vi "Configure Trigger (LIN).vi"(0 "VISA resource name":refnum<visa-resource-name>, 5 "Trigger Source (9: Bus 1)":u16(ring)=9 items=["Bus 1"=9, "Bus 2"=10, "Bus 3"=11, "Bus 4"=12], 7 "Condition (0: Sync field)":u16(ring) items=["Sync Field", "Identifier", "Data", "ID and data", "Wake up", "Sleep", "Error"], 9 "Data":T1={"Data Size (8)"=8, "Data Value (XXXXXXXX)"="XXXXXXXX", "Data Upper Word Value (XXXXXXXX)"="XXXXXXXX", "Data Qualifier (0: Less than)"=0, "Error Type (0: Sync)"=0, "Identifier Value (XXXXXXXX)"="XXXXXXXX"} {"Error Type (0: Sync)" items=["Sync", "Parity", "Checksum", "Header time", "Response time", "Frame time"]; "Data Qualifier (0: Less than)" items=["Less than", "More than", "Equal", "Unequal", "Less equal", "More equal", "In range", "Out of range"]}, 11 "error in (no error)":errorcluster) -> (4 "VISA resource name out":refnum<visa-resource-name>, 15 "error out":errorcluster)   [LabVIEW 2017, in "Scope.lvlib" / "Tektronix DPO MSO 2000 4000 Series.lvlib"]
doc: "Configures Audio trigger settings for an oscilloscope."
uses:
  Tektronix DPO MSO 2000 4000 Series.lvlib
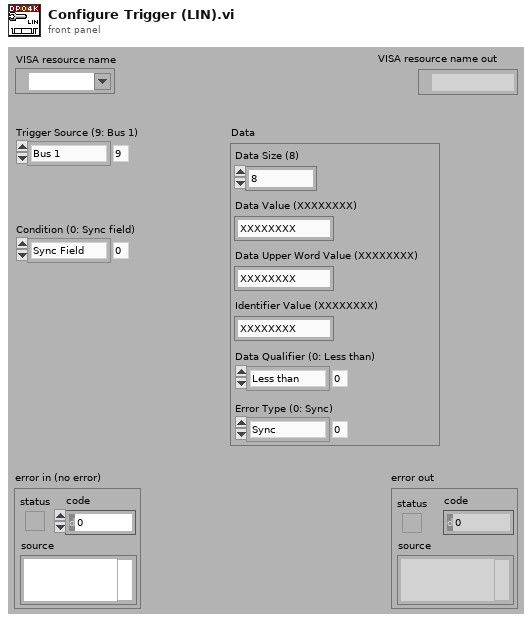
[diagram p1: front panel]
types:
  T1 = cluster{"Data Size (8)":i32, "Data Value (XXXXXXXX)":string, "Data Upper Word Value (XXXXXXXX)":string, "Data Qualifier (0: Less than)":u16, "Error Type (0: Sync)":u16, "Identifier Value (XXXXXXXX)":string}
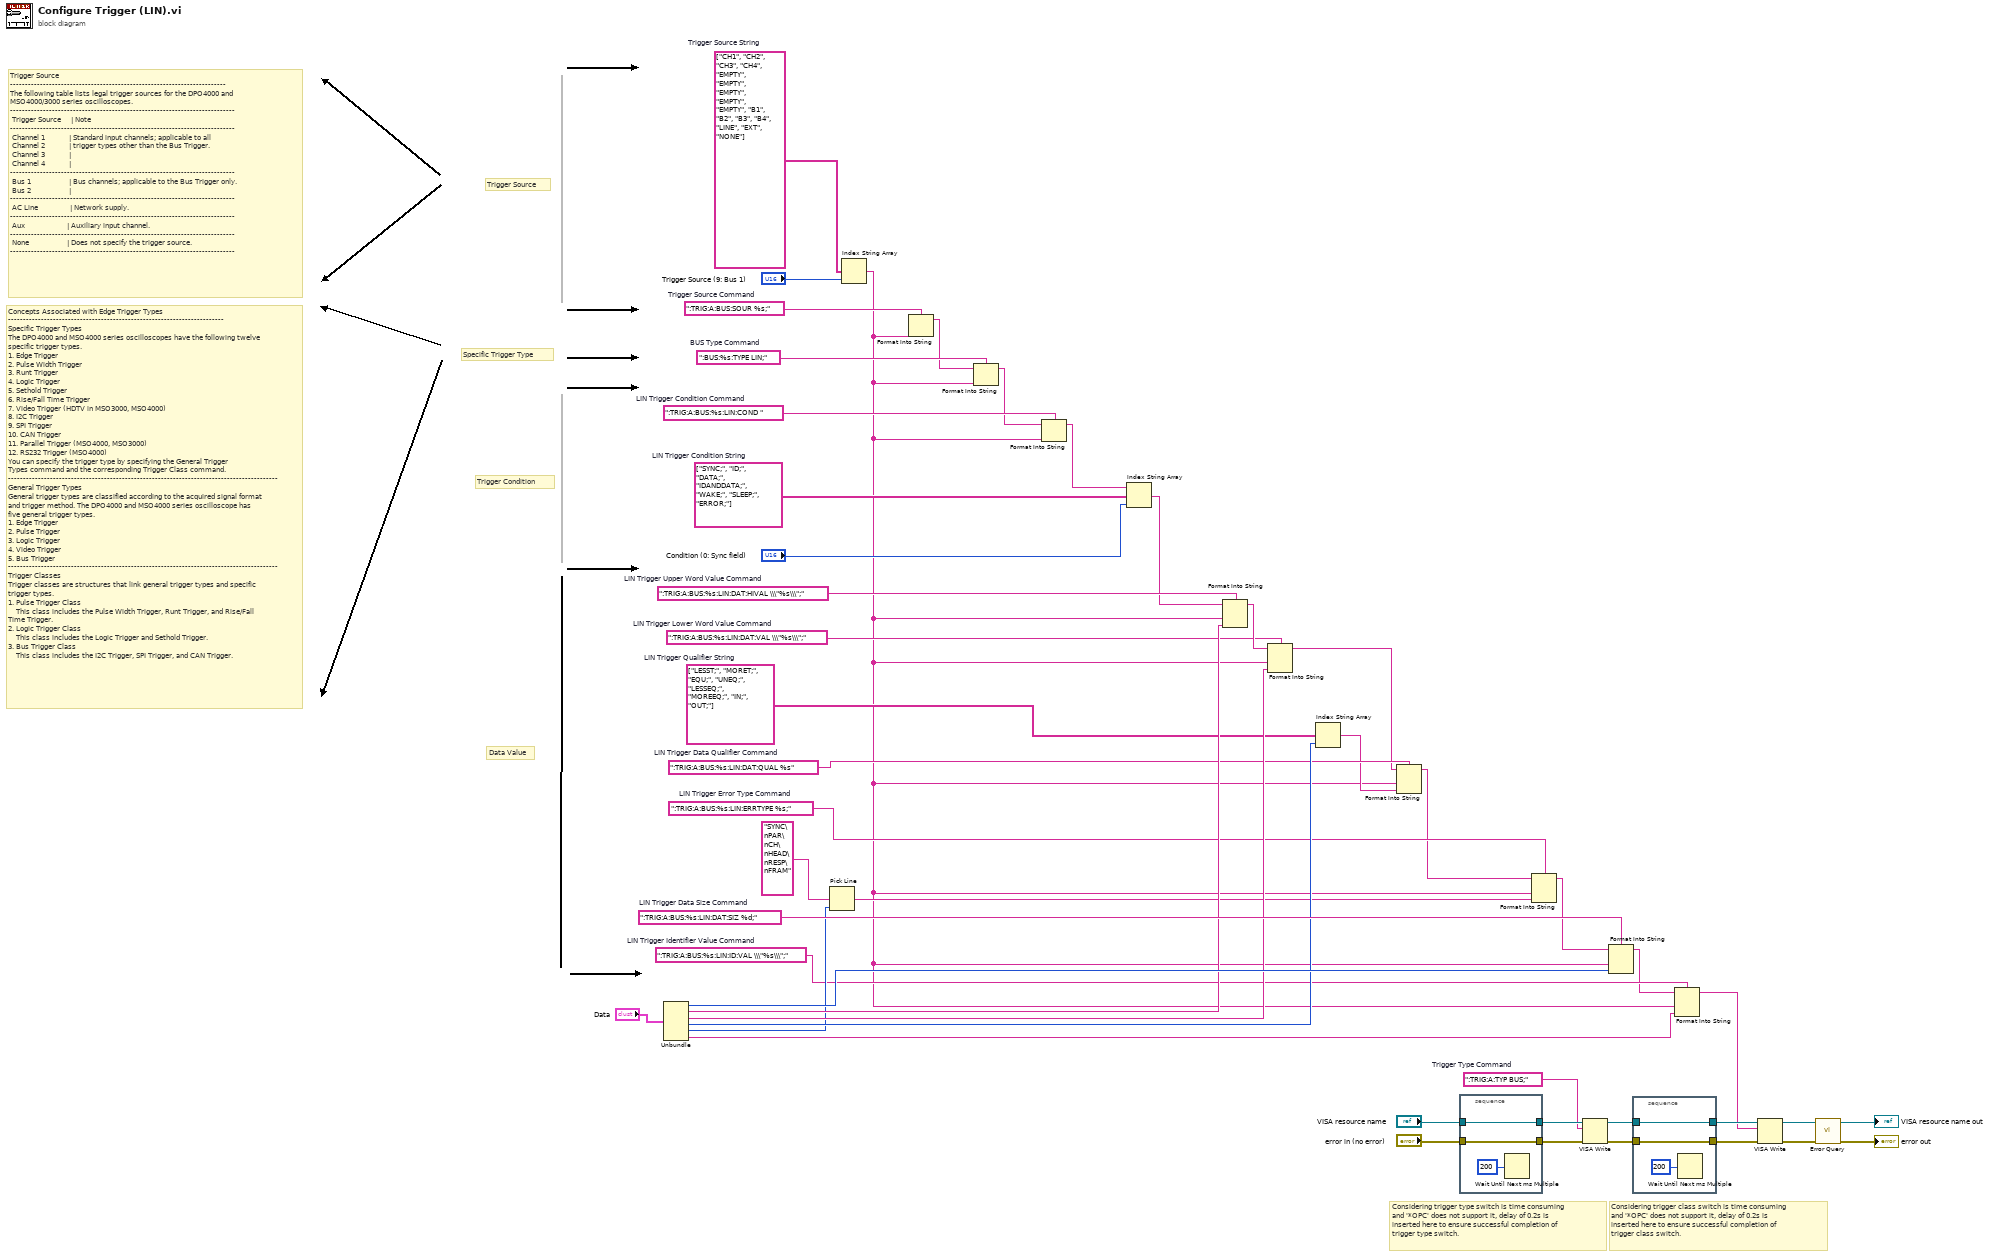
[diagram p0: block diagram]
diagram:
  w5 = ":TRIG:A:BUS:%s:LIN:ID:VAL \\\"%s\\\";"  # LIN Trigger Identifier Value Command
  w8 = ":TRIG:A:BUS:%s:LIN:ERRTYPE %s;"  # LIN Trigger Error Type Command
  w13 = ":TRIG:A:BUS:%s:LIN:DAT:QUAL %s"  # LIN Trigger Data Qualifier Command
  w15 = string[] ["LESST;", "MORET;", "EQU;", "UNEQ;", "LESSEQ;", "MOREEQ;", "IN;", "OUT;"]  # LIN Trigger Qualifier String
  w17 = ":TRIG:A:BUS:%s:LIN:DAT:VAL \\\"%s\\\";"  # LIN Trigger Lower Word Value Command
  w29 = string[] ["CH1", "CH2", "CH3", "CH4", "EMPTY", "EMPTY", "EMPTY", "EMPTY", "EMPTY", "B1", "B2", "B3", "B4", "LINE", "EXT", "NONE"]  # Trigger Source String
  w28 = ":TRIG:A:BUS:SOUR %s;"  # Trigger Source Command
  w36 = ":TRIG:A:TYP BUS;"  # Trigger Type Command
  w42 = ":TRIG:A:BUS:%s:LIN:DAT:SIZ %d;"  # LIN Trigger Data Size Command
  w43 = ":TRIG:A:BUS:%s:LIN:DAT:HIVAL \\\"%s\\\";"  # LIN Trigger Upper Word Value Command
  w45 = string[] ["SYNC;", "ID;", "DATA;", "IDANDDATA;", "WAKE;", "SLEEP;", "ERROR;"]  # LIN Trigger Condition String
  w47 = ":TRIG:A:BUS:%s:LIN:COND "  # LIN Trigger Condition Command
  w27 = ":BUS:%s:TYPE LIN;"  # BUS Type Command
  # "Concepts Associated with Edge Trigger Types\n------------------------------------------------------------------------\nSpecific Trigger Types\nThe DPO4000 and MSO4000 series oscilloscopes have the following twelve specific trigger types.\n1. Edge Trigger\n2. Pulse Width Trigger\n3. Runt Trigger\n4. Logic Trigger\n5. Sethold Trigger\n6. Rise/Fall Time Trigger\n7. Video Trigger (HDTV in MSO3000, MSO4000)\n8. I2C Trigger\n9. SPI Trigger\n10. CAN Trigger\n11. Parallel Trigger (MSO4000, MSO3000)\n12. RS232 Trigger (MSO4000)\nYou can specify the trigger type by specifying the General Trigger \nTypes command and the corresponding Trigger Class command.\n------------------------------------------------------------------------------------------\nGeneral Trigger Types \nGeneral trigger types are classified according to the acquired signal format and trigger method. The DPO4000 and MSO4000 series oscilloscope has five general trigger types.\n1. Edge Trigger\n2. Pulse Trigger\n3. Logic Trigger\n4. Video Trigger\n5. Bus Trigger\n------------------------------------------------------------------------------------------\nTrigger Classes\nTrigger classes are structures that link general trigger types and specific trigger types.\n1. Pulse Trigger Class\n    This class includes the Pulse Width Trigger, Runt Trigger, and Rise/Fall Time Trigger.\n2. Logic Trigger Class\n    This class includes the Logic Trigger and Sethold Trigger.\n3. Bus Trigger Class\n    This class includes the I2C Trigger, SPI Trigger, and CAN Trigger."
  # "Trigger Source\n------------------------------------------------------------------------\nThe following table lists legal trigger sources for the DPO4000 and MSO4000/3000 series oscilloscopes.\n---------------------------------------------------------------------------\n Trigger Source     | Note                                                           \n---------------------------------------------------------------------------\n Channel 1            | Standard input channels; applicable to all      \n Channel 2            | trigger types other than the Bus Trigger.         \n Channel 3            |     \n Channel 4            |\n---------------------------------------------------------------------------\n Bus 1                   | Bus channels; applicable to the Bus Trigger only.\n Bus 2                   | \n---------------------------------------------------------------------------\n AC Line                | Network supply.\n---------------------------------------------------------------------------\n Aux                     | Auxiliary input channel.\n---------------------------------------------------------------------------\n None                   | Does not specify the trigger source.\n---------------------------------------------------------------------------"
  # "Data Value"
  # "Trigger Condition"
  # "Specific Trigger Type"
  # "Trigger Source"
  # "Considering trigger class switch is time consuming\nand '*OPC' does not support it, delay of 0.2s is \ninserted here to ensure successful completion of\ntrigger class switch."
  # "Considering trigger type switch is time consuming\nand '*OPC' does not support it, delay of 0.2s is \ninserted here to ensure successful completion of\ntrigger type switch."
  n1 = Unbundle("Data") -> ("Data Size (8)"=w39:i32, "Data Value (XXXXXXXX)"=w19:string, "Data Upper Word Value (XXXXXXXX)"=w16:string, "Data Qualifier (0: Less than)"=w14:u16, "Error Type (0: Sync)"=w9:u16, "Identifier Value (XXXXXXXX)"=w3:string)
  n2 = Pick Line(multi-line string="SYNC\nPAR\nCH\nHEAD\nRESP\nFRAM", line index=w9) -> (output string=w7:string)  [unwired: 1 in]
  n3 = Index String Array(1:"Trigger Source (9: Bus 1)", 2:w29) -> (0:w4:string)  [unwired: 1 in]
  n4 = Format Into String(format string=w28, w4) -> (resulting string=w24:string)  [unwired: 2 in, 1 out]
  n5 = Format Into String(format string=w27, initial string=w24, w4) -> (resulting string=w26:string)  [unwired: 1 in, 1 out]
  n6 = Format Into String(format string=w47, initial string=w26, w4) -> (resulting string=w46:string)  [unwired: 1 in, 1 out]
  n7 = Index String Array(1:"Condition (0: Sync field)", 2:w45, 3:w46) -> (0:w25:string)
  n8 = Format Into String(format string=w43, initial string=w25, w4, w19) -> (resulting string=w18:string)  [unwired: 1 in, 1 out]
  n9 = Format Into String(format string=w17, initial string=w18, w4, w16) -> (resulting string=w11:string)  [unwired: 1 in, 1 out]
  n10 = Index String Array(1:w14, 2:w15) -> (0:w12:string)  [unwired: 1 in]
  n11 = Format Into String(format string=w13, initial string=w11, w4, w12) -> (resulting string=w6:string)  [unwired: 1 in, 1 out]
  n12 = stacked-sequence {
    tunnel: "VISA resource name" -> [w50]
    tunnel: [w50] -> w38
    tunnel: "error in (no error)" -> [w49]
    tunnel: [w49] -> w37
    frame #0 {
      n13 = Wait Until Next ms Multiple(millisecond multiple=u32 200) -> ()  [unwired: 1 out]
    }
  }
  n14 = Format Into String(format string=w8, initial string=w6, w4, w7) -> (resulting string=w41:string)  [unwired: 1 in, 1 out]
  n15 = VISA Write(VISA resource name=w38, write buffer=w36, error in (no error)=w37) -> (VISA resource name out=w35:refnum<visa-resource-name>, error out=w34:errorcluster)  [unwired: 1 out]
  n16 = Format Into String(format string=w42, initial string=w41, w4, w39) -> (resulting string=w2:string)  [unwired: 1 in, 1 out]
  n17 = stacked-sequence {
    tunnel: w35 -> [w53]
    tunnel: [w53] -> w30
    tunnel: w34 -> [w52]
    tunnel: [w52] -> w33
    frame #0 {
      n18 = Wait Until Next ms Multiple(millisecond multiple=u32 200) -> ()  [unwired: 1 out]
    }
  }
  n19 = Format Into String(format string=w5, initial string=w2, w4, w3) -> (resulting string=w1:string)  [unwired: 1 in, 1 out]
  n20 = VISA Write(VISA resource name=w30, write buffer=w1, error in (no error)=w33) -> (VISA resource name out=w32:refnum<visa-resource-name>, error out=w31:errorcluster)  [unwired: 1 out]
  n21 = call "Error Query.vi"("error in (no error)"=w31, "VISA resource name"=w32) -> ("error out"=→"error out":errorcluster, "VISA resource name out"=→"VISA resource name out":refnum<visa-resource-name>)  [unwired: 6 in, 2 out]
